vi "RelayControl.vi"(2 "NHR or Battery Analyzer":enum16{"Battery Analyzer", "Power Supply"}(ring), 3 "Battery Select":T1(ring)) -> ()   [LabVIEW 2020]
uses:
  <vilib>/DAQmx/write.llb/DAQmx Write (Digital 1D Bool NChan 1Samp 1Line).vi
  <vilib>/DAQmx/read.llb/DAQmx Read (Analog 1D DBL NChan 1Samp).vi
  <vilib>/DAQmx/miscellaneous.llb/DAQmx Fill In Error Info.vi
panel:
  out "error out 2":errorcluster
  out "error out":errorcluster
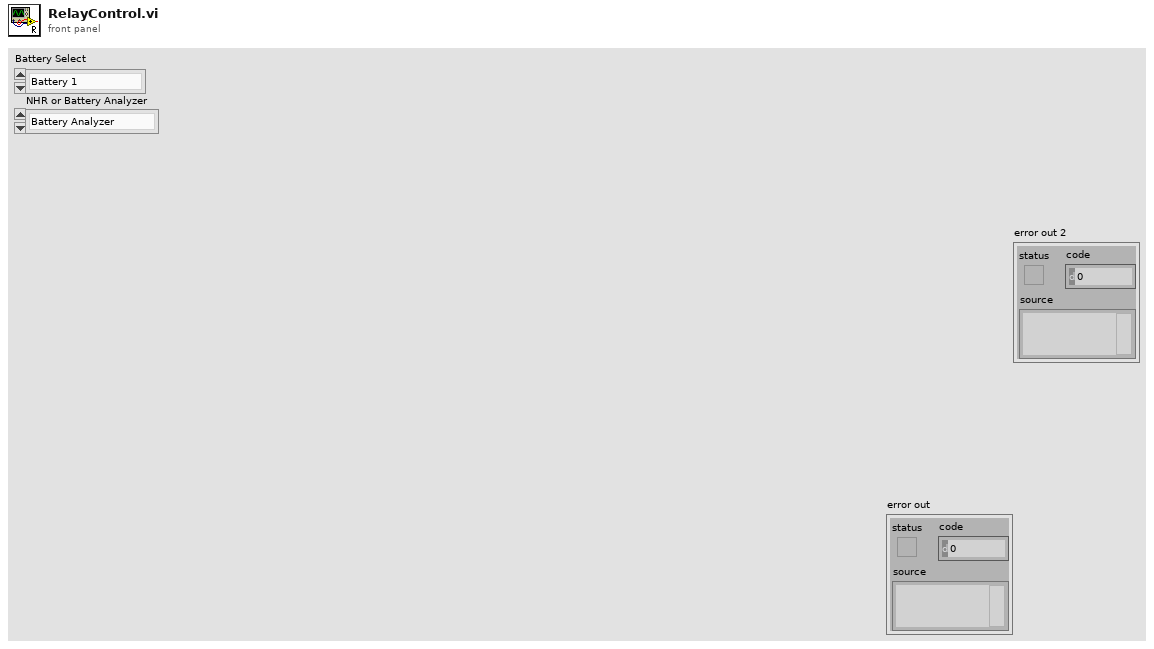
[diagram p1: front panel]
types:
  T1 = enum16{"Battery 1", "Battery 2", "Battery 3", "Battery 1&2", "Battery 1&3", "Battery 2&3", "Battery 1&2&3"}
  T2 = cluster{bool, bool, bool, bool, bool, bool, bool, bool, bool, bool, bool}
  T3 = cluster{"data[0]":dbl, "data[1]":dbl, "data[2]":dbl, "data[3]":dbl, "data[4]":dbl, "data[5]":dbl, "data[6]":dbl, "data[7]":dbl, "data[8]":dbl, "data[9]":dbl, "data[10]":dbl, "data[11]":dbl, "data[12]":dbl}
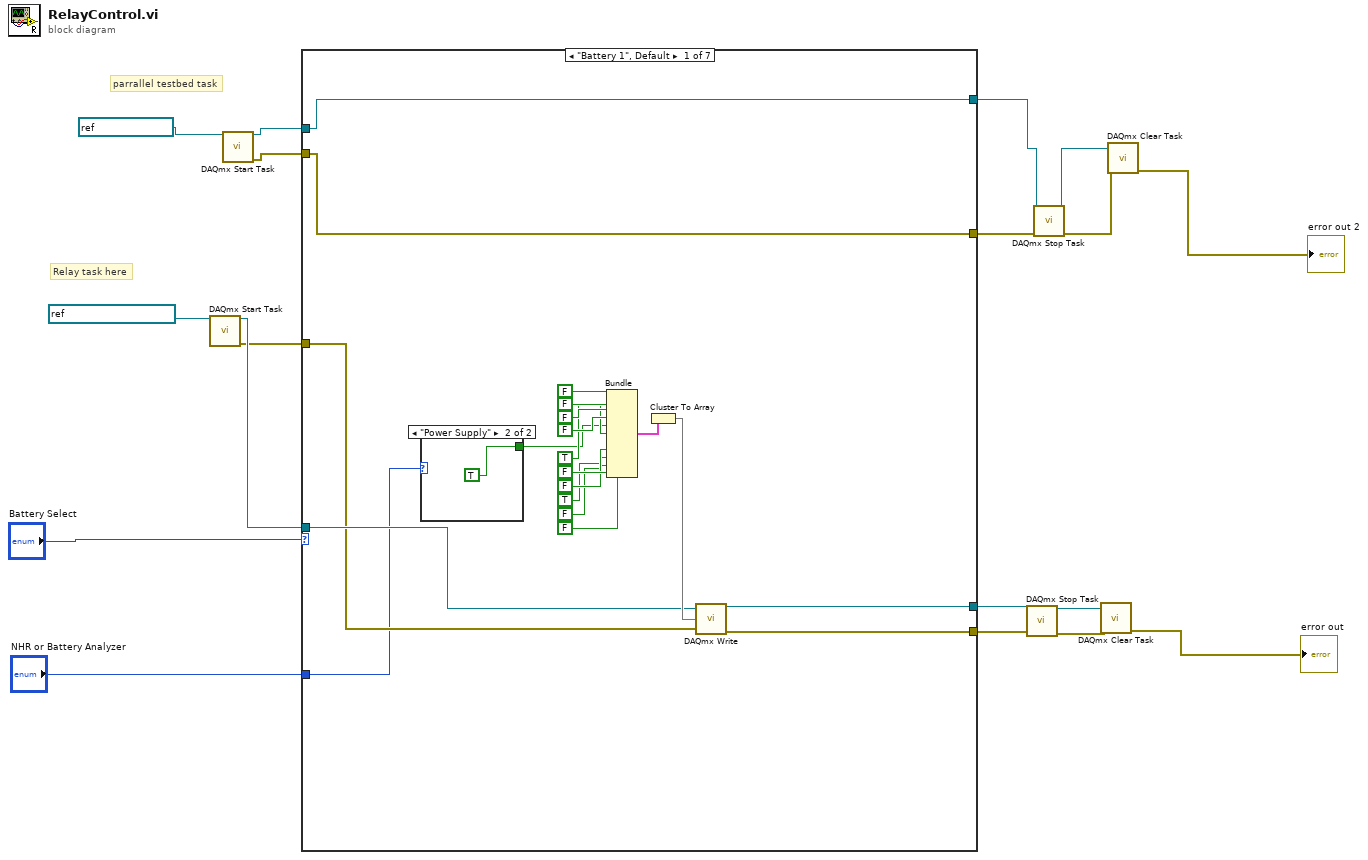
[diagram p0: block diagram]
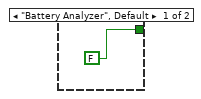
[diagram p2: hidden frame]
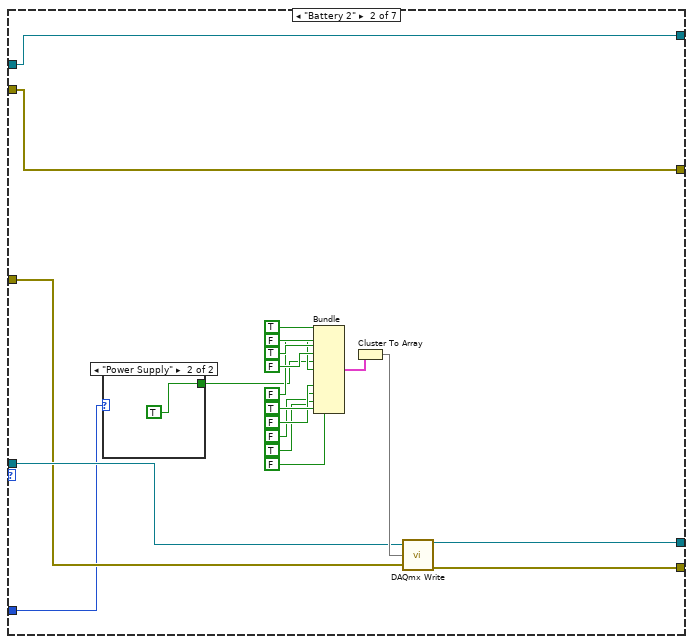
[diagram p3: hidden frame]
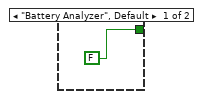
[diagram p4: hidden frame]
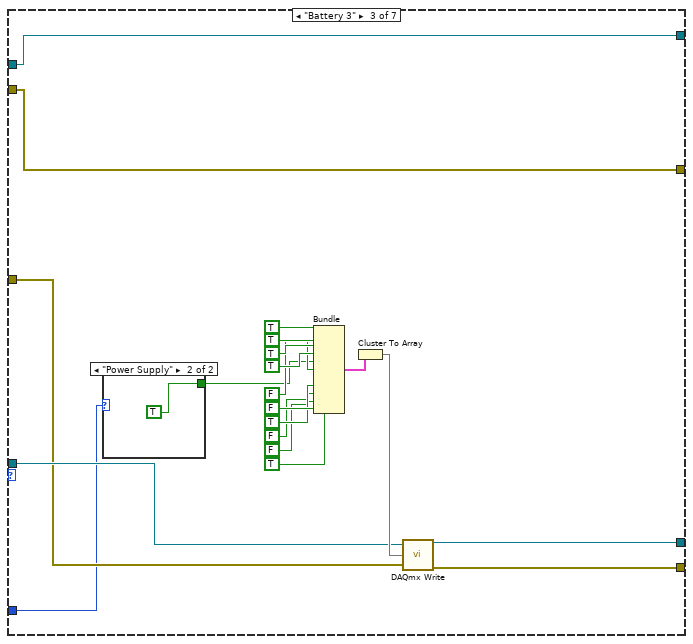
[diagram p5: hidden frame]
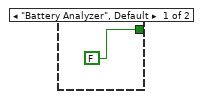
[diagram p6: hidden frame]
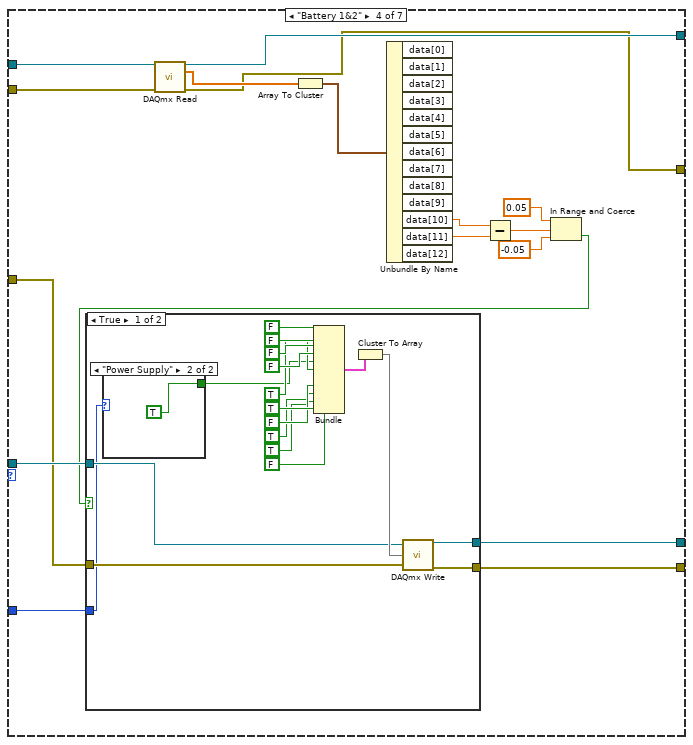
[diagram p7: hidden frame]
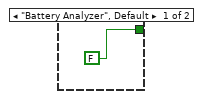
[diagram p8: hidden frame]
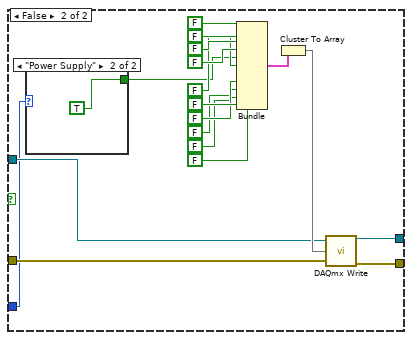
[diagram p9: hidden frame]
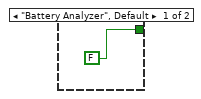
[diagram p10: hidden frame]
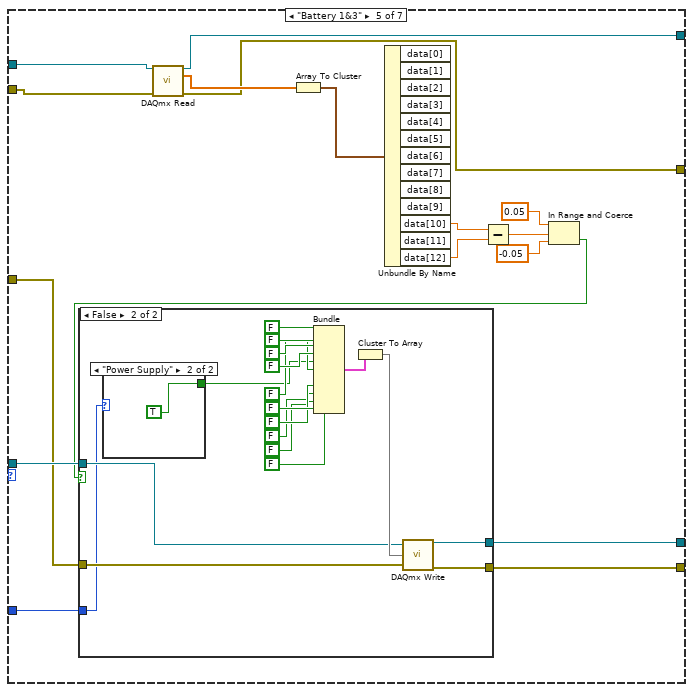
[diagram p11: hidden frame]
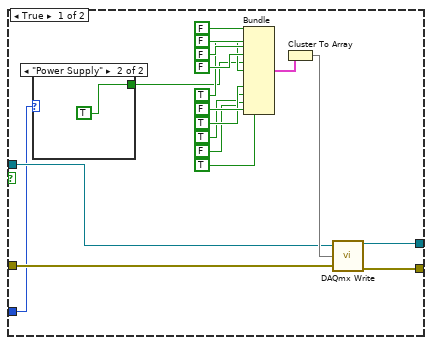
[diagram p12: hidden frame]
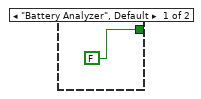
[diagram p13: hidden frame]
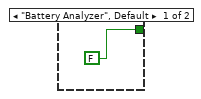
[diagram p14: hidden frame]
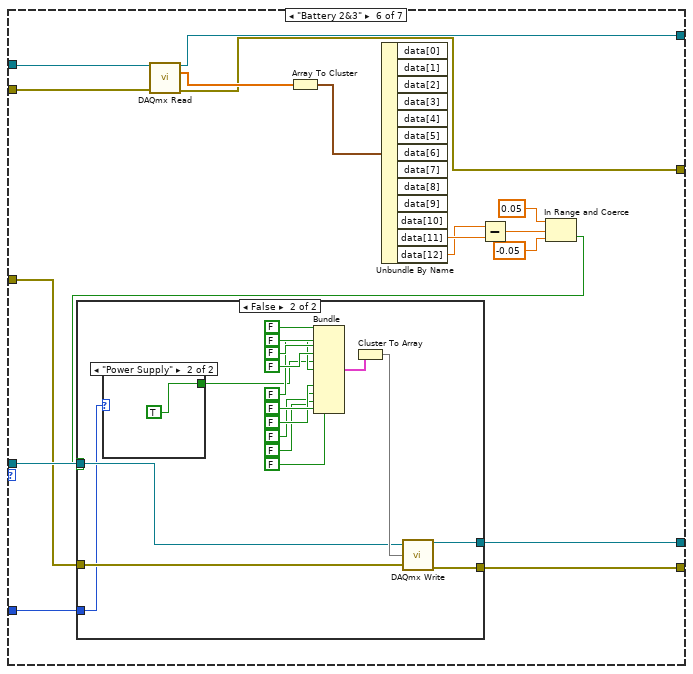
[diagram p15: hidden frame]
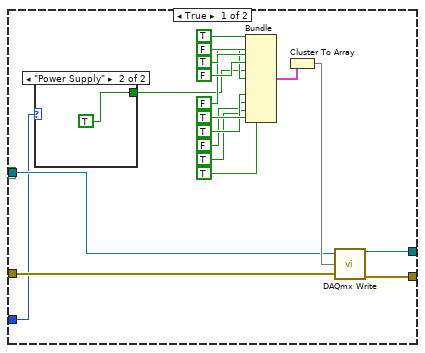
[diagram p16: hidden frame]
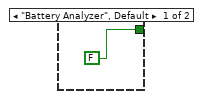
[diagram p17: hidden frame]
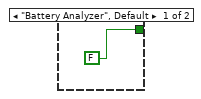
[diagram p18: hidden frame]
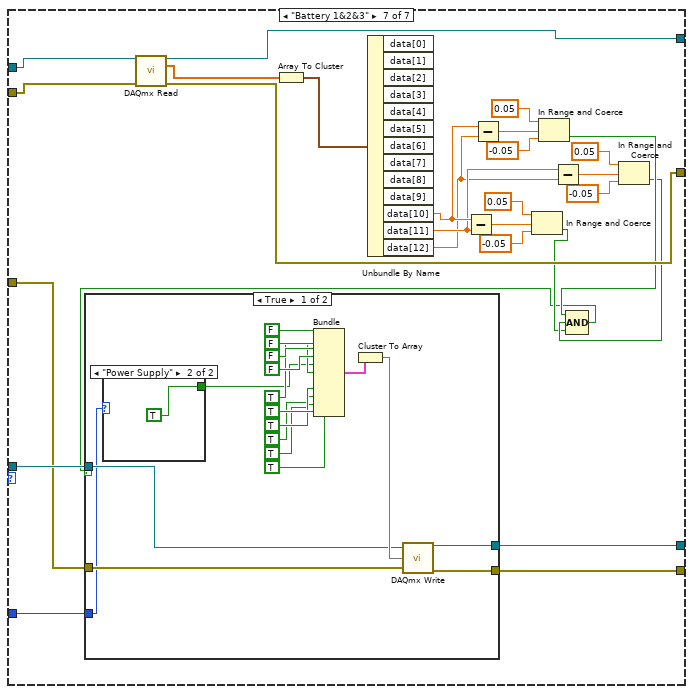
[diagram p19: hidden frame]
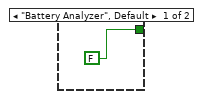
[diagram p20: hidden frame]
diagram:
  # "parrallel testbed task"
  # "Relay task here"
  n1 = call <vilib>:"DAQmx Start Task.vi"("task/channels in"=refnum<k21> "PTestbedRelayTask") -> ("task out"=w17:refnum<k21>, "error out"=w16:errorcluster)  [unwired: 13 in]
  n2 = call <vilib>:"DAQmx Start Task.vi"("task/channels in"=refnum<k21> "PTesbedTask") -> ("task out"=w7:refnum<k21>, "error out"=w6:errorcluster)  [unwired: 13 in]
  n3 = case shown="\"Battery 1\", Default" "Battery Select" {
    tunnel: w17 -> [w26 w48 w70 w101 w158 w215 w282]
    tunnel: w16 -> [w25 w47 w69 w100 w157 w214 w281]
    tunnel: "NHR or Battery Analyzer" -> [w24 w46 w68 w99 w156 w213 w280]
    tunnel: [w22 w44 w66 w98 w155 w212 w279] -> w11
    tunnel: [w21 w43 w65 w97 w154 w211 w278] -> w10
    tunnel: w7 -> [w20 w42 w64 w95 w146 w204 w272]
    tunnel: w6 -> [w19 w41 w63 w94 w145 w203 w271]
    tunnel: [w20 w42 w64 w93 w144 w202 w270] -> w2
    tunnel: [w19 w41 w63 w92 w143 w201 w269] -> w1
    frame "Battery 1", Default {
      n4 = case shown="\"Power Supply\"" w24 {
        tunnel: [FALSE TRUE] -> w23
        frame "Battery Analyzer", Default {
        }
        frame "Power Supply" {
        }
      }
      n5 = Bundle(FALSE, FALSE, FALSE, FALSE, w23, TRUE, FALSE, FALSE, TRUE, FALSE, FALSE) -> (w38:T2)  [unwired: 1 in]
      n6 = Cluster To Array(cluster=w38) -> (array=w31:bool[])
      n7 = call-poly <vilib>:"DAQmx Write.vi"("task/channels in"=w26, "data"=w31, "error in"=w25) -> ("task out"=w22:refnum<k21>, "error out"=w21:errorcluster)  [unwired: 10 in, 1 out]
    }
    frame "Battery 2" {
      n8 = case shown="\"Power Supply\"" w46 {
        tunnel: [FALSE TRUE] -> w45
        frame "Battery Analyzer", Default {
        }
        frame "Power Supply" {
        }
      }
      n9 = Bundle(TRUE, FALSE, TRUE, FALSE, w45, FALSE, TRUE, FALSE, FALSE, TRUE, FALSE) -> (w60:T2)  [unwired: 1 in]
      n10 = Cluster To Array(cluster=w60) -> (array=w53:bool[])
      n11 = call-poly <vilib>:"DAQmx Write.vi"("task/channels in"=w48, "data"=w53, "error in"=w47) -> ("task out"=w44:refnum<k21>, "error out"=w43:errorcluster)  [unwired: 10 in, 1 out]
    }
    frame "Battery 3" {
      n12 = case shown="\"Power Supply\"" w68 {
        tunnel: [FALSE TRUE] -> w67
        frame "Battery Analyzer", Default {
        }
        frame "Power Supply" {
        }
      }
      n13 = Bundle(TRUE, TRUE, TRUE, TRUE, w67, FALSE, FALSE, TRUE, FALSE, FALSE, TRUE) -> (w82:T2)  [unwired: 1 in]
      n14 = Cluster To Array(cluster=w82) -> (array=w75:bool[])
      n15 = call-poly <vilib>:"DAQmx Write.vi"("task/channels in"=w70, "data"=w75, "error in"=w69) -> ("task out"=w66:refnum<k21>, "error out"=w65:errorcluster)  [unwired: 10 in, 1 out]
    }
    frame "Battery 1&2" {
      n16 = call-poly <vilib>:"DAQmx Read.vi"("task/channels in"=w95, "error in"=w94) -> ("task out"=w93:refnum<k21>, "data"=w96:dbl[], "error out"=w92:errorcluster)  [unwired: 11 in]
      n17 = Array To Cluster(array=w96) -> (cluster=w88:T3)
      n18 = Unbundle By Name(w88) -> ("data[10]"=w87:dbl, "data[11]"=w86:dbl)  [unwired: 11 out]
      n19 = Subtract(x=w87, y=w86) -> (x-y=w91:dbl)
      n20 = In Range and Coerce(upper limit=0.05, x=w91, lower limit=-0.05) -> (In Range?=w85:bool)  [unwired: 1 out]
      n21 = case shown="True" w85 {
        tunnel: w101 -> [w107 w127]
        tunnel: w100 -> [w106 w126]
        tunnel: w99 -> [w105 w125]
        tunnel: [w103 w123] -> w98
        tunnel: [w102 w122] -> w97
        frame True {
          n22 = case shown="\"Power Supply\"" w105 {
            tunnel: [FALSE TRUE] -> w104
            frame "Battery Analyzer", Default {
            }
            frame "Power Supply" {
            }
          }
          n23 = Bundle(FALSE, FALSE, FALSE, FALSE, w104, TRUE, TRUE, FALSE, TRUE, TRUE, FALSE) -> (w119:T2)  [unwired: 1 in]
          n24 = Cluster To Array(cluster=w119) -> (array=w112:bool[])
          n25 = call-poly <vilib>:"DAQmx Write.vi"("task/channels in"=w107, "data"=w112, "error in"=w106) -> ("task out"=w103:refnum<k21>, "error out"=w102:errorcluster)  [unwired: 10 in, 1 out]
        }
        frame False {
          n26 = case shown="\"Power Supply\"" w125 {
            tunnel: [FALSE TRUE] -> w124
            frame "Battery Analyzer", Default {
            }
            frame "Power Supply" {
            }
          }
          n27 = Bundle(FALSE, FALSE, FALSE, FALSE, w124, FALSE, FALSE, FALSE, FALSE, FALSE, FALSE) -> (w139:T2)  [unwired: 1 in]
          n28 = Cluster To Array(cluster=w139) -> (array=w132:bool[])
          n29 = call-poly <vilib>:"DAQmx Write.vi"("task/channels in"=w127, "data"=w132, "error in"=w126) -> ("task out"=w123:refnum<k21>, "error out"=w122:errorcluster)  [unwired: 10 in, 1 out]
        }
      }
    }
    frame "Battery 1&3" {
      n30 = call-poly <vilib>:"DAQmx Read.vi"("task/channels in"=w146, "error in"=w145) -> ("task out"=w144:refnum<k21>, "data"=w153:dbl[], "error out"=w143:errorcluster)  [unwired: 11 in]
      n31 = Array To Cluster(array=w153) -> (cluster=w149:T3)
      n32 = Unbundle By Name(w149) -> ("data[10]"=w148:dbl, "data[12]"=w147:dbl)  [unwired: 11 out]
      n33 = Subtract(x=w148, y=w147) -> (x-y=w152:dbl)
      n34 = In Range and Coerce(upper limit=0.05, x=w152, lower limit=-0.05) -> (In Range?=w142:bool)  [unwired: 1 out]
      n35 = case shown="False" w142 {
        tunnel: w158 -> [w164 w184]
        tunnel: w157 -> [w163 w183]
        tunnel: w156 -> [w162 w182]
        tunnel: [w160 w180] -> w155
        tunnel: [w159 w179] -> w154
        frame True {
          n36 = case shown="\"Power Supply\"" w162 {
            tunnel: [FALSE TRUE] -> w161
            frame "Battery Analyzer", Default {
            }
            frame "Power Supply" {
            }
          }
          n37 = Bundle(FALSE, FALSE, FALSE, FALSE, w161, TRUE, FALSE, TRUE, TRUE, FALSE, TRUE) -> (w176:T2)  [unwired: 1 in]
          n38 = Cluster To Array(cluster=w176) -> (array=w169:bool[])
          n39 = call-poly <vilib>:"DAQmx Write.vi"("task/channels in"=w164, "data"=w169, "error in"=w163) -> ("task out"=w160:refnum<k21>, "error out"=w159:errorcluster)  [unwired: 10 in, 1 out]
        }
        frame False {
          n40 = case shown="\"Power Supply\"" w182 {
            tunnel: [FALSE TRUE] -> w181
            frame "Battery Analyzer", Default {
            }
            frame "Power Supply" {
            }
          }
          n41 = Bundle(FALSE, FALSE, FALSE, FALSE, w181, FALSE, FALSE, FALSE, FALSE, FALSE, FALSE) -> (w196:T2)  [unwired: 1 in]
          n42 = Cluster To Array(cluster=w196) -> (array=w189:bool[])
          n43 = call-poly <vilib>:"DAQmx Write.vi"("task/channels in"=w184, "data"=w189, "error in"=w183) -> ("task out"=w180:refnum<k21>, "error out"=w179:errorcluster)  [unwired: 10 in, 1 out]
        }
      }
    }
    frame "Battery 2&3" {
      n44 = call-poly <vilib>:"DAQmx Read.vi"("task/channels in"=w204, "error in"=w203) -> ("task out"=w202:refnum<k21>, "data"=w210:dbl[], "error out"=w201:errorcluster)  [unwired: 11 in]
      n45 = Array To Cluster(array=w210) -> (cluster=w206:T3)
      n46 = Unbundle By Name(w206) -> ("data[11]"=w205:dbl, "data[12]"=w200:dbl)  [unwired: 11 out]
      n47 = Subtract(x=w200, y=w205) -> (x-y=w209:dbl)
      n48 = In Range and Coerce(upper limit=0.05, x=w209, lower limit=-0.05) -> (In Range?=w199:bool)  [unwired: 1 out]
      n49 = case shown="False" w199 {
        tunnel: w215 -> [w221 w241]
        tunnel: w214 -> [w220 w240]
        tunnel: w213 -> [w219 w239]
        tunnel: [w217 w237] -> w212
        tunnel: [w216 w236] -> w211
        frame True {
          n50 = case shown="\"Power Supply\"" w219 {
            tunnel: [FALSE TRUE] -> w218
            frame "Battery Analyzer", Default {
            }
            frame "Power Supply" {
            }
          }
          n51 = Bundle(TRUE, FALSE, TRUE, FALSE, w218, FALSE, TRUE, TRUE, FALSE, TRUE, TRUE) -> (w233:T2)  [unwired: 1 in]
          n52 = Cluster To Array(cluster=w233) -> (array=w226:bool[])
          n53 = call-poly <vilib>:"DAQmx Write.vi"("task/channels in"=w221, "data"=w226, "error in"=w220) -> ("task out"=w217:refnum<k21>, "error out"=w216:errorcluster)  [unwired: 10 in, 1 out]
        }
        frame False {
          n54 = case shown="\"Power Supply\"" w239 {
            tunnel: [FALSE TRUE] -> w238
            frame "Battery Analyzer", Default {
            }
            frame "Power Supply" {
            }
          }
          n55 = Bundle(FALSE, FALSE, FALSE, FALSE, w238, FALSE, FALSE, FALSE, FALSE, FALSE, FALSE) -> (w253:T2)  [unwired: 1 in]
          n56 = Cluster To Array(cluster=w253) -> (array=w246:bool[])
          n57 = call-poly <vilib>:"DAQmx Write.vi"("task/channels in"=w241, "data"=w246, "error in"=w240) -> ("task out"=w237:refnum<k21>, "error out"=w236:errorcluster)  [unwired: 10 in, 1 out]
        }
      }
    }
    frame "Battery 1&2&3" {
      n58 = call-poly <vilib>:"DAQmx Read.vi"("task/channels in"=w272, "error in"=w271) -> ("task out"=w270:refnum<k21>, "data"=w277:dbl[], "error out"=w269:errorcluster)  [unwired: 11 in]
      n59 = Array To Cluster(array=w277) -> (cluster=w273:T3)
      n60 = Unbundle By Name(w273) -> ("data[10]"=w262:dbl, "data[11]"=w261:dbl, "data[12]"=w260:dbl)  [unwired: 10 out]
      n61 = Subtract(x=w262, y=w261) -> (x-y=w276:dbl)
      n62 = Subtract(x=w262, y=w260) -> (x-y=w268:dbl)
      n63 = In Range and Coerce(upper limit=0.05, x=w276, lower limit=-0.05) -> (In Range?=w257:bool)  [unwired: 1 out]
      n64 = In Range and Coerce(upper limit=0.05, x=w268, lower limit=-0.05) -> (In Range?=w259:bool)  [unwired: 1 out]
      n65 = Subtract(x=w261, y=w260) -> (x-y=w265:dbl)
      n66 = In Range and Coerce(upper limit=0.05, x=w265, lower limit=-0.05) -> (In Range?=w258:bool)  [unwired: 1 out]
      n67 = Compound Arithmetic op=AND(w259, w258, w257) -> (w256:bool)
      n68 = case shown="True" w256 {
        tunnel: w282 -> [w288 w308]
        tunnel: w281 -> [w287 w307]
        tunnel: w280 -> [w286 w306]
        tunnel: [w284 w304] -> w279
        tunnel: [w283 w303] -> w278
        frame True {
          n69 = case shown="\"Power Supply\"" w286 {
            tunnel: [FALSE TRUE] -> w285
            frame "Battery Analyzer", Default {
            }
            frame "Power Supply" {
            }
          }
          n70 = Bundle(FALSE, FALSE, FALSE, FALSE, w285, TRUE, TRUE, TRUE, TRUE, TRUE, TRUE) -> (w300:T2)  [unwired: 1 in]
          n71 = Cluster To Array(cluster=w300) -> (array=w293:bool[])
          n72 = call-poly <vilib>:"DAQmx Write.vi"("task/channels in"=w288, "data"=w293, "error in"=w287) -> ("task out"=w284:refnum<k21>, "error out"=w283:errorcluster)  [unwired: 10 in, 1 out]
        }
        frame False {
          n73 = case shown="\"Power Supply\"" w306 {
            tunnel: [FALSE TRUE] -> w305
            frame "Battery Analyzer", Default {
            }
            frame "Power Supply" {
            }
          }
          n74 = Bundle(FALSE, FALSE, FALSE, FALSE, w305, FALSE, FALSE, FALSE, FALSE, FALSE, FALSE) -> (w320:T2)  [unwired: 1 in]
          n75 = Cluster To Array(cluster=w320) -> (array=w313:bool[])
          n76 = call-poly <vilib>:"DAQmx Write.vi"("task/channels in"=w308, "data"=w313, "error in"=w307) -> ("task out"=w304:refnum<k21>, "error out"=w303:errorcluster)  [unwired: 10 in, 1 out]
        }
      }
    }
  }
  n77 = call <vilib>:"DAQmx Stop Task.vi"("task/channels in"=w11, "error in"=w10) -> ("task out"=w14:refnum<k21>, "error out"=w13:errorcluster)  [unwired: 12 in]
  n78 = call <vilib>:"DAQmx Stop Task.vi"("task/channels in"=w2, "error in"=w1) -> ("task out"=w5:refnum<k21>, "error out"=w4:errorcluster)  [unwired: 12 in]
  n79 = call <vilib>:"DAQmx Clear Task.vi"("task in"=w14, "error in"=w13) -> ("error out"=→"error out":errorcluster)  [unwired: 13 in]
  n80 = call <vilib>:"DAQmx Clear Task.vi"("task in"=w5, "error in"=w4) -> ("error out"=→"error out 2":errorcluster)  [unwired: 13 in]
